vi "CT_MatchCapNumWithLED.vi"(1 "Cap Module Number":i32[][](array[numeric])=[[43, 44, 45, 46, 47, 48, 0, 0, 0, 0], [33, 34, 35, 36, 37, 38, 39, 40, 41, 42], [71, 72, 25, 26, 27, 28, 29, 30, 31, 32], [61, 62, 63, 64, 65, 66, 67, 68, 69, 70], [51, 52, 53, 54, 55, 56, 57, 58, 59, 60], [49, 50, 92, 96, 17, 21, 20, 24, 89, 93], [1, 2, 3, 4, 5, 6, 7, 8, 73, 74], [75, 76, 77, 78, 79, 80, 81, 82, 83, 84], [9, 10, 11, 12, 13, 14, 15, 16, 18, 19], [22, 23, 85, 86, 87, 88, 90, 91, 94, 95]], 2 "Discharge Identity":string[][](array[string])) -> (0 "Formation=False":bool[][](array[boolean]))   [LabVIEW 2016]
panel:
  out "Array 2":string[](array[string])
  out "Array":string[](array[string])
  out "size(s)":i32[](array[numeric])
  out "subarray":i32[](array[numeric])
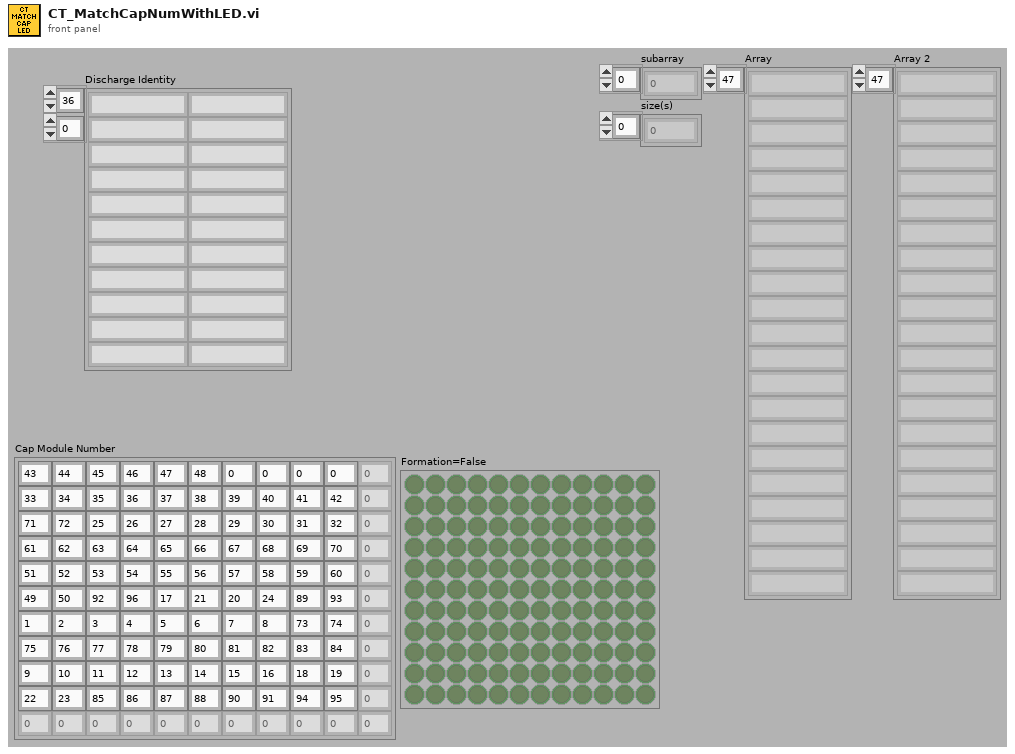
[diagram p1: front panel]
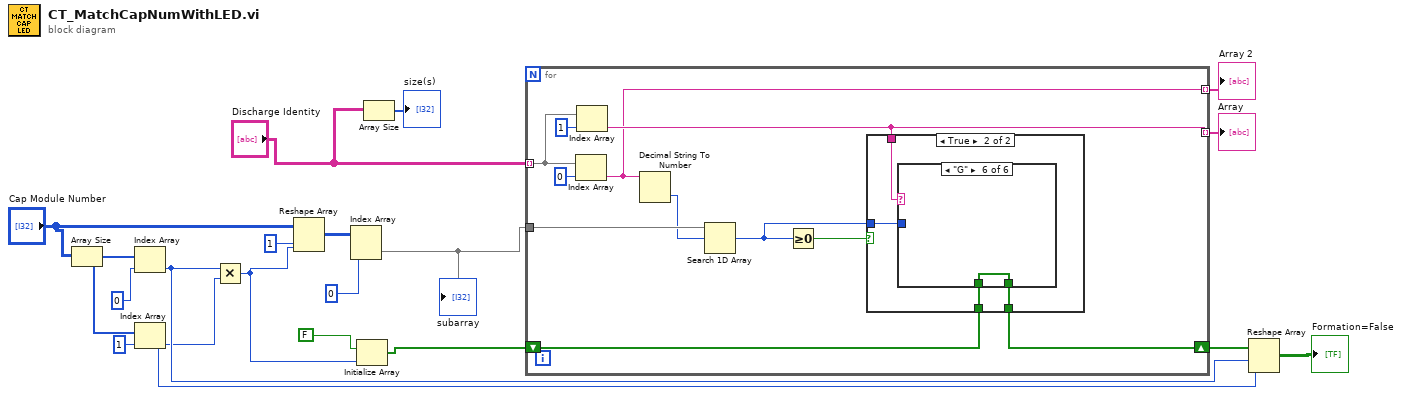
[diagram p0: block diagram]
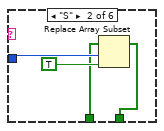
[diagram p4: hidden frame]
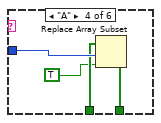
[diagram p6: hidden frame]
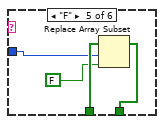
[diagram p7: hidden frame]
diagram:
  n1 = Array Size(array="Cap Module Number") -> (size(s)=w9:i32[])
  n2 = Index Array(array=w9, index=0 ("dimension size")) -> (element=w6:i32)
  n3 = Index Array(array=w9, index=1) -> (element=w5:i32)
  n4 = Multiply(x=w6, y=w5) -> (x*y=w7:i32)
  n5 = Reshape Array("Cap Module Number", 1, w7) -> (w18:i32[][])
  n6 = Index Array(array=w18, index (row)=0) -> (element=w16:i32[])  [unwired: 1 in]
  "subarray" <- w16
  n7 = Initialize Array(FALSE, w7) -> (w14:bool[])
  n8 = Array Size(array="Discharge Identity") -> (size(s)=→"size(s)":i32[])
  n9 = for {
    tunnel: w16 -> [w30]
    tunnel: "Discharge Identity" -> [w26] mode=indexing
    shift-right: [w23] -> w13
    shift-left: w14 -> [w22]
    tunnel: [w21] -> w2 mode=indexing
    tunnel: [w20] -> w1 mode=indexing
    n10 = Index Array(array=w26, index=0) -> (element=w20:string)
    n11 = Index Array(array=w26, index=1) -> (element=w21:string)
    n12 = Decimal String To Number(string=w20) -> (number=w28:i32)  [unwired: 2 in, 1 out]
    n13 = Search 1D Array(1D array=w30, element=w28) -> (index of element=w25:i32)  [unwired: 1 in]
    n14 = Greater Or Equal To 0?(x=w25) -> (x >= 0?=w24:bool)
    n15 = case shown="True" w24 {
      tunnel: w25 -> [_ w35]
      tunnel: w21 -> [_ w34]
      tunnel: w22 -> [w31 w33]
      tunnel: [w31 w32] -> w23
      frame False {
      }
      frame True {
        n16 = case shown="\"G\"" w34 {
          tunnel: w35 -> [_ w39 _ w45 w47 _]
          tunnel: w33 -> [w36 w37 w41 w44 w49 w50]
          tunnel: [w36 w38 w41 w42 w46 w50] -> w32
          frame Default {
          }
          frame "S" {
            n17 = Replace Array Subset(array=w37, new element=TRUE ("new element/subarray"), index=w39) -> (w38:bool[])
          }
          frame "D" {
          }
          frame "A" {
            n18 = Replace Array Subset(array=w44, new element=TRUE ("new element/subarray"), index=w45) -> (w42:bool[])
          }
          frame "F" {
            n19 = Replace Array Subset(array=w49, new element=FALSE ("new element/subarray"), index=w47) -> (w46:bool[])
          }
          frame "G" {
          }
        }
      }
    }
  }
  "Array" <- w2
  "Array 2" <- w1
  n20 = Reshape Array(w13, w6, w5) -> (→"Formation=False":bool[][])
